vi "CalcMotorSpeed.vi"(8 "Reference Voltage (12)":dbl=12.0, 9 "Motor Characteristics":T1, 10 "Motor Torque":dbl, 11 "Motor Voltage":dbl) -> (3 "Motor Speed":dbl)   [LabVIEW 2014]
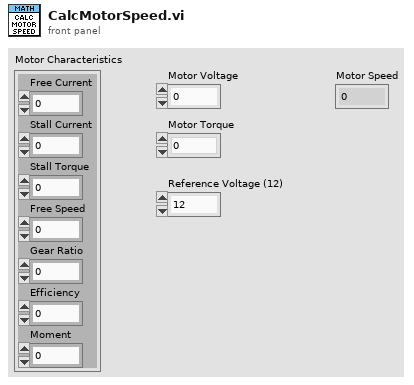
[diagram p1: front panel]
types:
  T1 = cluster{"Free Current":dbl, "Stall Current":dbl, "Stall Torque":dbl, "Free Speed":dbl, "Gear Ratio":dbl, "Efficiency":dbl, "Moment":dbl}
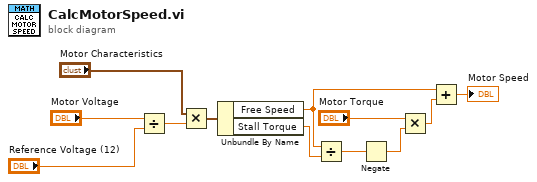
[diagram p0: block diagram]
diagram:
  n1 = Divide(x="Motor Voltage", y="Reference Voltage (12)") -> (x/y=w10:dbl)
  n2 = Multiply(x="Motor Characteristics", y=w10) -> (x*y=w8:T1)
  n3 = Unbundle By Name(w8) -> ("Free Speed"=w2:dbl, "Stall Torque"=w7:dbl)
  n4 = Divide(x=w2, y=w7) -> (x/y=w6:dbl)
  n5 = Negate(x=w6) -> (-x=w5:dbl)
  n6 = Multiply(x="Motor Torque", y=w5) -> (x*y=w3:dbl)
  n7 = Add(x=w2, y=w3) -> (x+y=→"Motor Speed":dbl)
